vi "ELVIS III v1.0 RPC Unregister Heart Beat.vi"(8 "error in (no error)":errorcluster, 10 "Channel Names":string[](array[string]), 11 "Session":u32) -> (0 "error out":errorcluster)   [LabVIEW 2021]
uses:
  <vilib>/myRIO/Common/Instrument Driver Framework/ELVIS III v1.0/Resource Manager/typedefs/ELVIS III v1.0 RIO Session Map Action.ctl
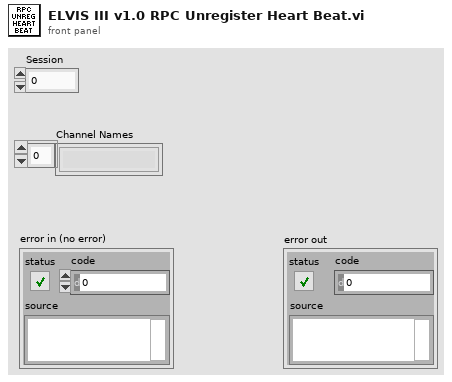
[diagram p1: front panel]
types:
  T1 = typedef "ELVIS III v1.0 RIO Session Map Action.ctl" = enum16{"Add Session", "Remove Session", "Get Active Sessions", "Get Owning Sessions"}
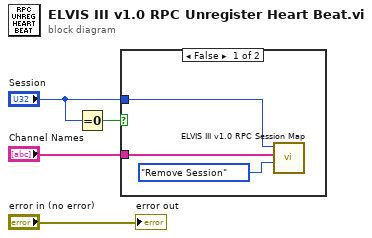
[diagram p0: block diagram]
diagram:
  n1 = Equal To 0?(x="Session") -> (x = 0?=w1:bool)
  n2 = case shown="False" w1 {
    tunnel: "Session" -> [w7 _]
    tunnel: "Channel Names" -> [w6 _]
    frame False {
      n3 = call <vilib>:"ELVIS III v1.0 RPC Session Map.vi"("Action"=ELVIS_III_v1.0_RIO_Session_Map_Action."Remove Session" ("Session Map Action"), "Channel Names"=w6, "Session"=w7) -> ()  [unwired: 7 in, 2 out]
    }
    frame True {
      # "Session is invalid i.e. call from rpc server"
    }
  }
  "error out" <- "error in (no error)"
